vi "Subvi AO trigger 20180614.vi"(10 "Ext trigger":bool) -> (2 "Scan direction":bool)   [LabVIEW 2017]
uses:
  <vilib>/Platform/TimedLoop/XDataNode/timing_clust.ctl
  <vilib>/Platform/TimedLoop/XDataNode/nitl_modes.ctl
  <vilib>/Platform/TimedLoop/XDataNode/wakeup.ctl
  <vilib>/rvi/Emulation/niFpgaSctlEmulationGetInTimedLoop.vi
  <vilib>/rvi/Emulation/niFpgaEmulationReportErrorSimple.vi
  <vilib>/rvi/Emulation/niFpgaGetClockAttributes.vi
  <vilib>/rvi/Emulation/niFpgaCriticalErrorInLSC.vi
  Detector/GV preframeclock.vi
  GV trigger delay.vi
  Detector/GV frame counter.vi
  <vilib>/Platform/TimedLoop/XDataNode/XDataNode.xnode
  <vilib>/Platform/TimedLoop/XDataNode/XDNodeRunTimeDep.lvlib
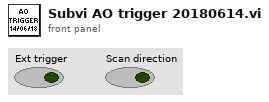
[diagram p1: front panel]
types:
  T1 = typedef "XDNodeRunTimeDep.lvlib/timing_clust.ctl" = cluster{"Expected End [f-1]":u64, "Actual End [f-1]":u64, "Finished Late? [f-1]":bool, "Expected End [i-1]":u64, "Actual End [i-1]":u64, "Finished Late? [i-1]":bool, "Expected Start [i]":u64, "Actual Start [i]":u64, "Expected Start [f]":u64, "Actual Start [f]":u64, "Source Name":string, "Structure Name":string, "Period":i64, "Deadline":i64, "Offset":i64, "Start":i64, "Priority":i32, "Timeout":i32, "Mode":T2, "Wakeup Reason":T3, "Error":errorcluster, "Source Type":string, "Secondary Source Type":string, "Global End Time":u64, "Global Start Time":u64, "Frame Duration":u64, "Iteration Duration":u64, "Assigned CPU":i32, "I/O Scan Engine Mode":u32}
  T2 = typedef "XDNodeRunTimeDep.lvlib/nitl_modes.ctl" = enum32{"No Change", "Process missed periods, maintain original phase", "Discard missed periods, maintain original phase", "Process missed periods, ignore original phase", "Discard missed periods, ignore original phase"}
  T3 = typedef "XDNodeRunTimeDep.lvlib/wakeup.ctl" = enum32{"Normal", "Aborted", "Asynchronous wakeup", "Timing source error", "Timed loop error", "Timeout"}
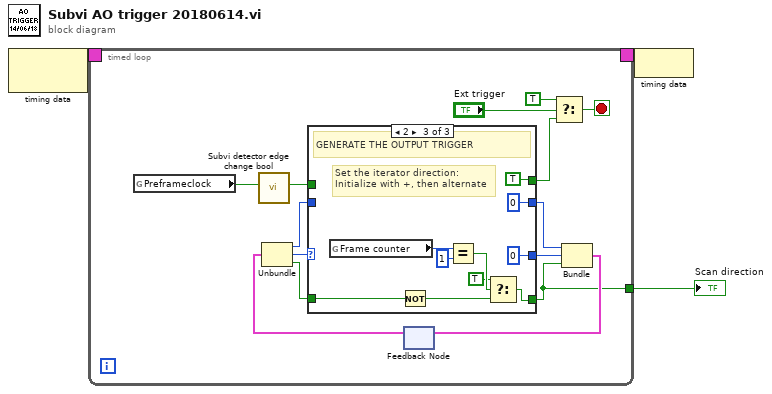
[diagram p0: block diagram]
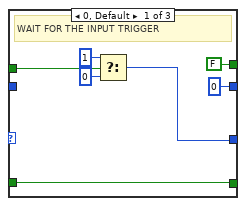
[diagram p2: hidden frame]
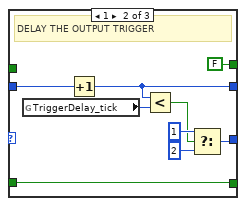
[diagram p3: hidden frame]
diagram:
  n1 = node-c288() -> (w3:T1)  [unwired: 1 in]
  n2 = timed-loop {
    timing: w3 -> [_]
    timing-out: [_] -> w2
    tunnel: [w6] -> w1
    stop <- w17 stop-if-true
    n3 = global read "GV preframeclock.vi" "Preframeclock"() -> (w5:bool)
    n4 = call "Subvi detector edge change bool.vi"("Input"=w5) -> ("Output"=w4:bool)  [unwired: 8 in]
    n5 = feedback #1() -> (w11:cluster{u16, "f":u8, bool})  [unwired: 1 in]
    n6 = Unbundle(w11) -> (w10:u16, "f"=w8:u8, w7:bool)
    n7 = case shown="2" w8 {
      tunnel: [u16 0 w31 u16 0] -> w14
      tunnel: [w24 w27 u8 0 ("f")] -> w9
      tunnel: w10 -> [_ w32 _]
      tunnel: [FALSE FALSE TRUE] -> w13
      tunnel: [w19 w25 w34] -> w6
      tunnel: w7 -> [w19 w25 w36]
      tunnel: w4 -> [w18 _ _]
      frame 0, Default {
        # "WAIT FOR THE INPUT TRIGGER"
        n8 = Select(t=u8 1, s=w18, f=u8 0) -> (s? t:f=w24:u8)
      }
      frame 1 {
        # "DELAY THE OUTPUT TRIGGER"
        n9 = global read "GV trigger delay.vi" "TriggerDelay_tick"() -> (w33:u16)
        n10 = Increment(x=w32) -> (x+1=w31:u16)
        n11 = Less?(x=w31, y=w33) -> (x < y?=w29:bool)
        n12 = Select(t=u8 1, s=w29, f=u8 2) -> (s? t:f=w27:u8)
      }
      frame 2 {
        # "Set the iterator direction:\nInitialize with +, then alternate"
        # "GENERATE THE OUTPUT TRIGGER"
        n13 = global read "GV frame counter.vi" "Frame counter"() -> (w38:u8)
        n14 = Not(x=w36) -> (.not. x?=w35:bool)
        n15 = Equal?(x=w38, y=u8 1) -> (x = y?=w40:bool)
        n16 = Select(t=TRUE, s=w40, f=w35) -> (s? t:f=w34:bool)
      }
    }
    n17 = Select(t=TRUE, s="Ext trigger", f=w13) -> (s? t:f=w17:bool)
    n18 = Bundle(w14, "f"=w9, w6) -> (w12:cluster{u16, "f":u8, bool})  [unwired: 1 in]
    n19 = feedback-in #1(w12) -> ()
  }
  "Scan direction" <- w1
  n20 = node-c288(w2) -> ()
